vi "ADS1115_READ_SINGLE_SAMPLE.vi"(7 "Scale Value (mV)":dbl=2.0, 8 "error in (no error)":errorcluster, 9 "options_i2c_read":T1, 10 "I2C Slave Address (0)":u8, 11 "handle":u32) -> (0 "error out":errorcluster, 1 "mV out":dbl, 2 "Data":u8[](array[numeric]), 3 "handle out":u32, 4 "x << y":u16, 5 "(hi.lo)":u16)   [LabVIEW 2017]
uses:
  libMPSSE.lvlib
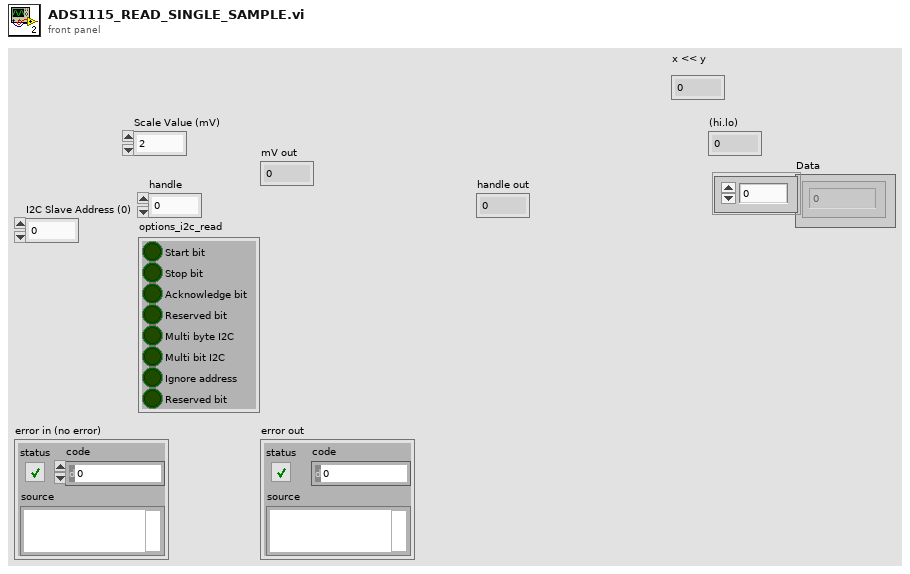
[diagram p1: front panel]
types:
  T1 = cluster{"Start bit":bool, "Stop bit":bool, "Acknowledge bit":bool, "Reserved bit":bool, "Multi byte I2C":bool, "Multi bit I2C":bool, "Ignore address":bool, "Reserved bit":bool}
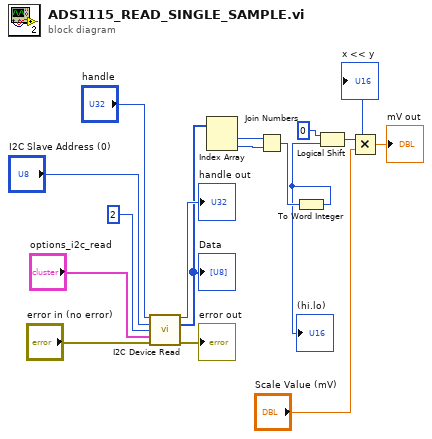
[diagram p0: block diagram]
diagram:
  n1 = call "I2C Device Read.vi"("handle"="handle", "Slave device address"="I2C Slave Address (0)", "Size to transfer"=u8 2 ("Bytes To Read"), "options"="options_i2c_read", "error in (no error)"="error in (no error)") -> ("handle out"=→"handle out":u32, "Data read"=w6:u8[], "error out"=→"error out":errorcluster)  [unwired: 6 in, 2 out]
  "Data" <- w6
  n2 = Index Array(array=w6) -> (element #1=w13:u8, element #2=w14:u8)  [unwired: 2 in]
  n3 = Join Numbers(hi=w13, lo=w14) -> ((hi.lo)=w2:u16)
  n4 = To Word Integer(number=w2) -> (16bit integer=w1:i16)
  "(hi.lo)" <- w1
  n5 = Logical Shift(y=i8 0, x=w1) -> (x << y=w15:i16)
  "x << y" <- w15
  n6 = Multiply(x=w15, y="Scale Value (mV)") -> (x*y=→"mV out":dbl)
